vi "Acquire and Read Frames.vi"(7 "additional timeout, ms (0)":u32, 8 "error in (no error)":errorcluster, 11 "SOL Camera in":refnum<class "PL SOL Instruments Camera.lvclass">) -> (0 "error out":errorcluster, 2 "frames":cluster{u16[]}[][](array[cluster]), 3 "SOL Camera out":refnum<class "PL SOL Instruments Camera.lvclass">)   [LabVIEW 2015, in "PL SOL Instruments Camera.lvclass"]
doc: "Acquires and reads frames."
uses:
  PL SOL Instruments Camera.lvclass
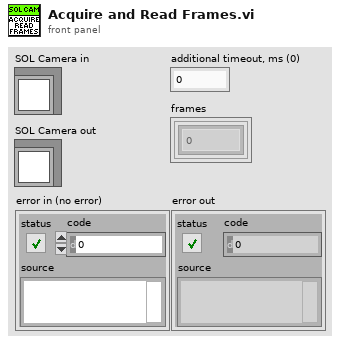
[diagram p1: front panel]
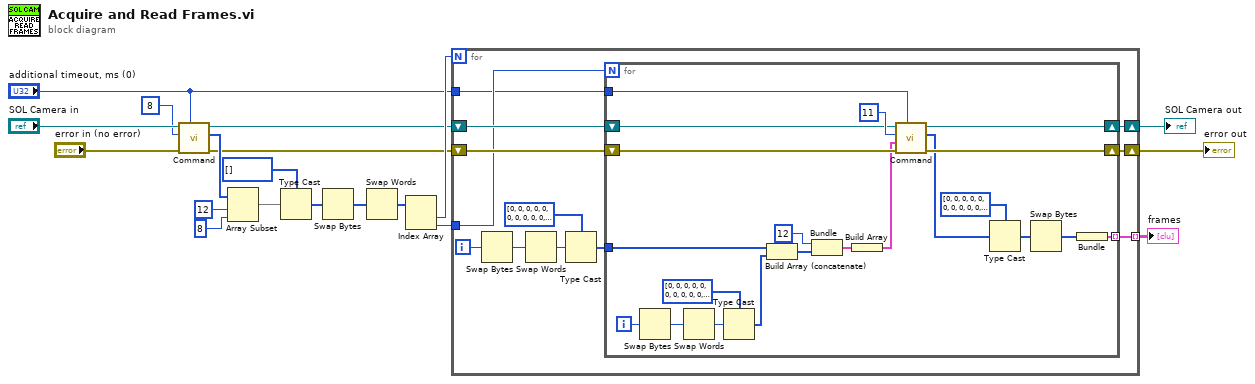
[diagram p0: block diagram]
diagram:
  n1 = call "Command.vi"("additional timeout, ms (0)"="additional timeout, ms (0)", "error in (no error)"="error in (no error)", "command"=u8 8, "SOL Camera in"="SOL Camera in") -> ("error out"=w1:errorcluster, "response"=w3:u8[], "SOL Camera out"=w6:refnum<class "PL SOL Instruments Camera.lvclass">)  [unwired: 5 in]
  n2 = Array Subset(array=w3, index=12, length=8 ("index")) -> (w17:u8[])
  n3 = Type Cast(type=i32[] [], x=w17) -> (*(type *) &x=w14:i32[])
  n4 = Swap Bytes(anything=w14) -> (byte swapped=w15:i32[])
  n5 = Swap Words(1:w15) -> (0:w13:i32[])
  n6 = Index Array(array=w13) -> (element #1=w10:i32, element #2=w9:i32)  [unwired: 2 in]
  n7 = for {
    N: w10 -> [_]
    shift-right: [w26] -> w5
    shift-left: w6 -> [w31]
    shift-right: [w25] -> w4
    shift-left: w1 -> [w24]
    tunnel: w9 -> [w22]
    tunnel: [w21] -> w7 mode=indexing
    tunnel: "additional timeout, ms (0)" -> [w20]
    i -> [w23]
    n8 = Swap Bytes(anything=w23) -> (byte swapped=w28:i32)
    n9 = Swap Words(1:w28) -> (0:w27:i32)
    n10 = Type Cast(type=u8[] [0, 0, 0, 0, 0, 0, 0, 0, 0, 0, 0, 0, 0, 0, 0, 0, 0, 0, 0, 0, 0, 0, 0, 0, 0, 0, 0, 0, 0, 0, 0, 0, 0, 0, 0, 0, 0, 0, 0, 0, 0, 0, 0, 0, 0, 0, 0, 0, 0, 0, 0, 0, 0, 0, 0, 0, 0, 0, 0, 0, 0, 0, 0, 0, 0, 0, 0, 0, 0, 0, 0, 0, 0, 0, 0, 0, 0, 0, 0, 0, 0, 0, 0, 0, 0, 0, 0, 0, 0, 0, 0, 0, 0, 0, 0, 0, 0, 0, 0, 0, 4, 0, 0, 0, 0, 0, 0, 0, 0, 0, 0, 0, 0, 0, 0, 0, 0, 0, 0, 0, 0, 0, 0, 0, 0, 0, 0, 0, 0, 0, 0, 0, 0, 0, 0, 0, 0, 0, 0, 0, 0, 0, 0, 0, 0, 0, 0, 0, 0, 0, 0, 0, 0, 0, 0, 0, 0, 0, 0, 0, 0, 0, 0, 0, 0, 0, 0, 0, 0, 0, 0, 0, 0, 0, 0, 0, 0, 0, 0, 0, 0, 0, 0, 0, 0, 0, 0, 0, 0, 0, 0, 0, 0, 0, 0, 0, 0, 0, 0, 0, 0, 0, 0, 0, 0, 0, 0, 0, 0, 0, 0, 0, 0, 0, 0, 0, 0, 0, 0, 0, 0, 0, 0, 0] ("response"), x=w27) -> (*(type *) &x=w29:u8[])
    n11 = for {
      N: w22 -> [_]
      tunnel: w29 -> [w50]
      tunnel: [w40] -> w21 mode=indexing
      shift-right: [w39] -> w26
      shift-left: w31 -> [w34]
      shift-right: [w38] -> w25
      shift-left: w24 -> [w36]
      tunnel: w20 -> [w32]
      i -> [w43]
      n12 = Swap Bytes(anything=w43) -> (byte swapped=w45:i32)
      n13 = Swap Words(1:w45) -> (0:w44:i32)
      n14 = Type Cast(type=u8[] [0, 0, 0, 0, 0, 0, 0, 0, 0, 0, 0, 0, 0, 0, 0, 0, 0, 0, 0, 0, 0, 0, 0, 0, 0, 0, 0, 0, 0, 0, 0, 0, 0, 0, 0, 0, 0, 0, 0, 0, 0, 0, 0, 0, 0, 0, 0, 0, 0, 0, 0, 0, 0, 0, 0, 0, 0, 0, 0, 0, 0, 0, 0, 0, 0, 0, 0, 0, 0, 0, 0, 0, 0, 0, 0, 0, 0, 0, 0, 0, 0, 0, 0, 0, 0, 0, 0, 0, 0, 0, 0, 0, 0, 0, 0, 0, 0, 0, 0, 0, 4, 0, 0, 0, 0, 0, 0, 0, 0, 0, 0, 0, 0, 0, 0, 0, 0, 0, 0, 0, 0, 0, 0, 0, 0, 0, 0, 0, 0, 0, 0, 0, 0, 0, 0, 0, 0, 0, 0, 0, 0, 0, 0, 0, 0, 0, 0, 0, 0, 0, 0, 0, 0, 0, 0, 0, 0, 0, 0, 0, 0, 0, 0, 0, 0, 0, 0, 0, 0, 0, 0, 0, 0, 0, 0, 0, 0, 0, 0, 0, 0, 0, 0, 0, 0, 0, 0, 0, 0, 0, 0, 0, 0, 0, 0, 0, 0, 0, 0, 0, 0, 0, 0, 0, 0, 0, 0, 0, 0, 0, 0, 0, 0, 0, 0, 0, 0, 0, 0, 0, 0, 0, 0, 0] ("response"), x=w44) -> (*(type *) &x=w41:u8[])
      n15 = Build Array (concatenate)(w50, w41) -> (w42:u8[])
      n16 = Bundle("offset"=12, w42) -> (w51:cluster{"offset":i32, u8[]})  [unwired: 1 in]
      n17 = Build Array(w51) -> (w35:cluster{"offset":i32, u8[]}[])
      n18 = call "Command.vi"("additional timeout, ms (0)"=w32, "error in (no error)"=w36, "data"=w35, "command"=u8 11, "SOL Camera in"=w34) -> ("error out"=w38:errorcluster, "response"=w33:u8[], "SOL Camera out"=w39:refnum<class "PL SOL Instruments Camera.lvclass">)  [unwired: 4 in]
      n19 = Type Cast(type=u16[] [0, 0, 0, 0, 0, 0, 0, 0, 0, 0, 0, 0, 0, 0, 0, 0, 0, 0, 0, 0, 0, 0, 0, 0, 0, 0, 0, 0, 0, 0, 0, 0, 0, 0, 0, 0, 0, 0, 0, 0, 0, 0, 0, 0, 0, 0, 0, 0, 0, 0, 0, 0, 0, 0, 0, 0, 0, 0, 0, 0, 0, 0, 0, 0, 0, 0, 0, 0, 0, 0, 0, 0, 0, 0, 0, 0, 0, 0, 0, 0, 0, 0, 0, 0, 0, 0, 0, 0, 0, 0, 0, 0, 0, 0, 0, 0, 0, 0, 0, 0, 4, 0, 0, 0, 0, 0, 0, 0, 0, 0, 0, 0, 0, 0, 0, 0, 0, 0, 0, 0, 0, 0, 0, 0, 0, 0, 0, 0, 0, 0, 0, 0, 0, 0, 0, 0, 0, 0, 0, 0, 0, 0, 0, 0, 0, 0, 0, 0, 0, 0, 0, 0, 0, 0, 0, 0, 0, 0, 0, 0, 0, 0, 0, 0, 0, 0, 0, 0, 0, 0, 0, 0, 0, 0, 0, 0, 0, 0, 0, 0, 0, 0, 0, 0, 0, 0, 0, 0, 0, 0, 0, 0, 0, 0, 0, 0, 0, 0, 0, 0, 0, 0, 0, 0, 0, 0, 0, 0, 0, 0, 0, 0, 0, 0, 0, 0, 0, 0, 0, 0, 0, 0, 0, 0] ("response"), x=w33) -> (*(type *) &x=w47:u16[])
      n20 = Swap Bytes(anything=w47) -> (byte swapped=w49:u16[])
      n21 = Bundle(w49) -> (w40:cluster{u16[]})  [unwired: 1 in]
    }
  }
  "SOL Camera out" <- w5
  "error out" <- w4
  "frames" <- w7
